vi "PCI1220U运行.vi"(9 "方向":u16, 11 "AxisHandle IN":u32) -> (3 "AxisHandle OUT":u32)   [LabVIEW 2013]
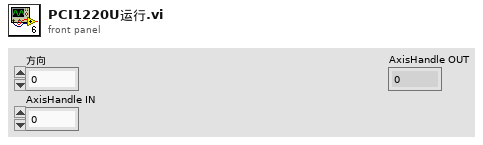
[diagram p1: front panel]
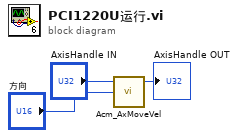
[diagram p0: block diagram]
diagram:
  n1 = call <userlib>:"Acm_AxMoveVel.vi"("Direction"="方向", "AxisHandle"="AxisHandle IN") -> ("AxisHandle"=→"AxisHandle OUT":u32)  [unwired: 1 in, 2 out]
